vi "Jog Move.vi"(4 "Stop Move":bool, 5 "Error In":errorcluster, 6 "Velocity [rev/s]":dbl(knob)=1000.0 scale=0.0..10.0, 7 "Position Limit [deg]":dbl=1000.0, 8 "Resource in":refnum<k21>="Axis 1") -> (0 "Move Position":dbl(graph), 1 "Jogging":bool, 2 "error out":errorcluster, 3 "Resource out":refnum<k21>="Axis 1")   [LabVIEW 2018]
uses:
  <vilib>/Motion/Express/_s/nimc.ex.clearFaults.clearFaults.axis.vi
  <vilib>/Motion/Express/_s/nimc.ex.read.readExecutionData.axis.vi
  <vilib>/Motion/Express/_s/nimc.ex.stopMove.stop.axis.modeDecelerate.vi
  <vilib>/Motion/Express/_s/nimc.ex.straightLineMove.startStraightLineMove.axis.modeAbsolute.0.vi
  <vilib>/Motion/BlockNode/FB.NIMotion.xnode
panel:
  out "Jog done":bool
  # "INPUTS"
  # "Stop Move"
  # "OUTPUTS"
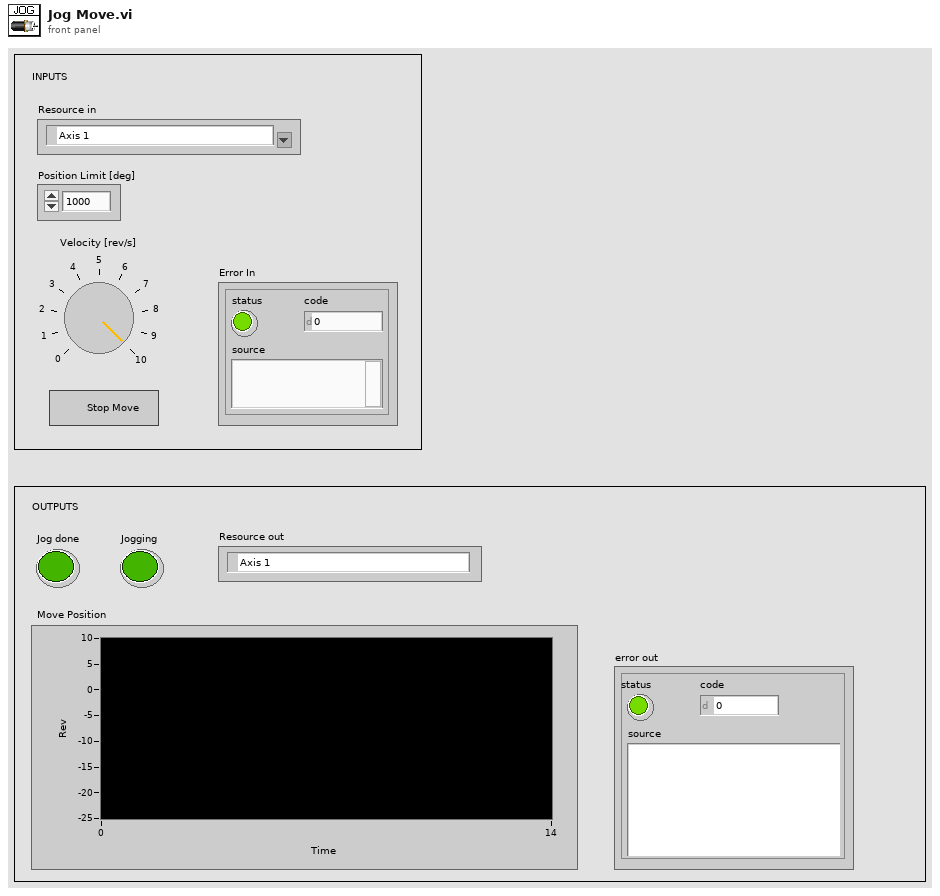
[diagram p1: front panel]
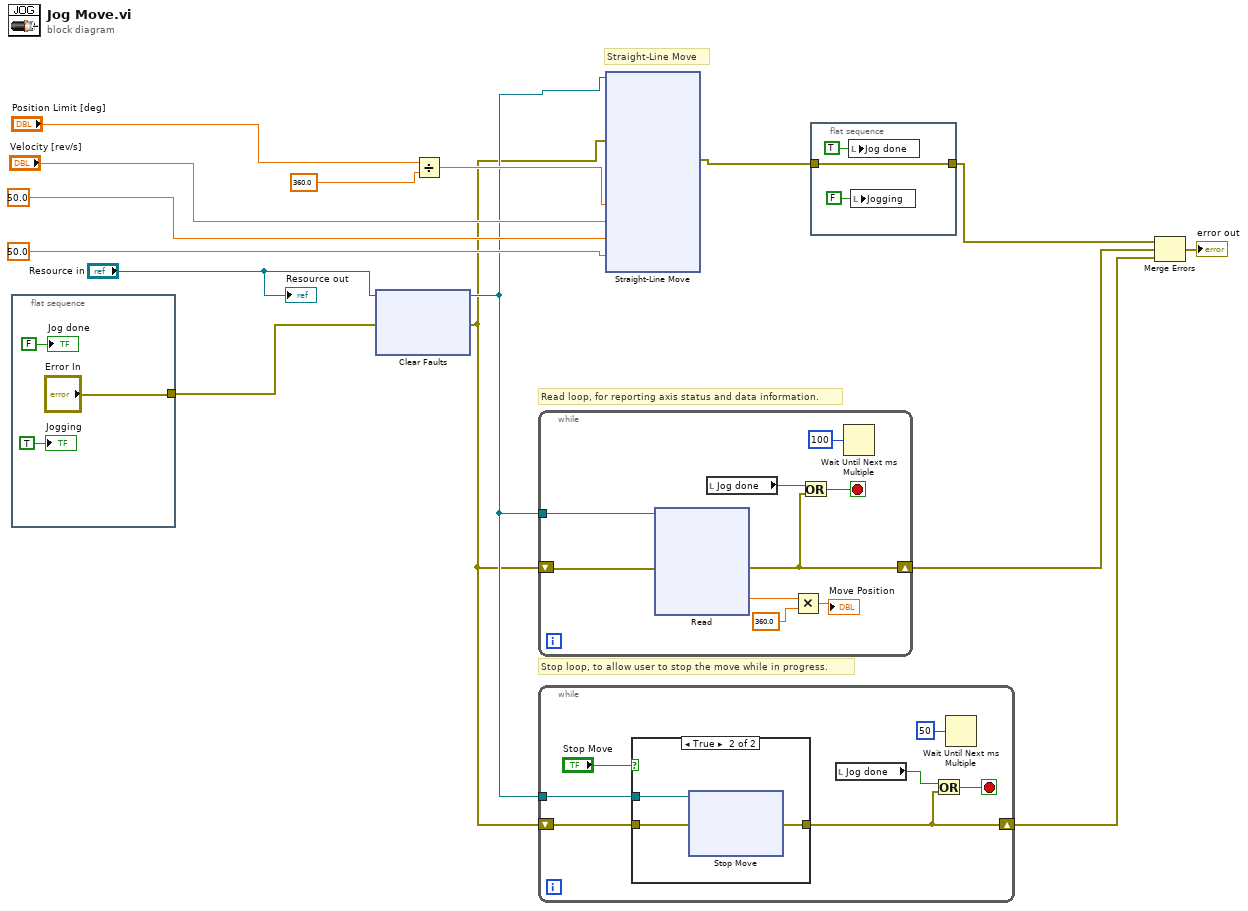
[diagram p0: block diagram]
diagram:
  # "Read loop, for reporting axis status and data information."
  # "Stop loop, to allow user to stop the move while in progress."
  # "Straight-Line Move"
  n1 = flat-sequence {
    tunnel: ["Error In"] -> w12
    frame #0 {
      "Jog done" <- FALSE ("Example Done")
      "Jogging" <- TRUE ("Example Done")
    }
  }
  n2 = xnode ("Clear Faults")("resource"="Resource in", "error in"=w12) -> ("resource out"=w4:refnum<k21>, "error out"=w1:errorcluster)
  n3 = Divide(x="Position Limit [deg]", y=360.0) -> (x/y=w5:dbl)
  n4 = while {
    tunnel: w4 -> [w25]
    shift-right: [w24] -> w14
    shift-left: w1 -> [w22]
    stop <- w27 stop-if-true
    n5 = xnode ("Read")("resource"=w25, "error in"=w22) -> ("position"=w21:dbl, "error out"=w24:errorcluster)  [unwired: 5 out]
    n6 = local read "Jog done"() -> (w26:bool)
    n7 = Multiply(x=w21, y=360.0) -> (x*y=→"Move Position":dbl)
    n8 = Or(x=w26, y=w24) -> (x .or. y?=w27:bool)
    n9 = Wait Until Next ms Multiple(millisecond multiple=u32 100) -> ()  [unwired: 1 out]
  }
  n10 = while {
    tunnel: w4 -> [w41]
    shift-right: [w39] -> w13
    shift-left: w1 -> [w40]
    stop <- w37 stop-if-true
    n11 = case shown="True" "Stop Move" {
      tunnel: [w44 w47] -> w39
      tunnel: w41 -> [_ w46]
      tunnel: w40 -> [w44 w45]
      frame False {
      }
      frame True {
        n12 = xnode ("Stop Move")("resource"=w46, "error in"=w45) -> ("error out"=w47:errorcluster)  [unwired: 1 in, 2 out]
      }
    }
    n13 = local read "Jog done"() -> (w38:bool)
    n14 = Or(x=w38, y=w39) -> (x .or. y?=w37:bool)
    n15 = Wait Until Next ms Multiple(millisecond multiple=u32 50) -> ()  [unwired: 1 out]
  }
  n16 = xnode ("Straight-Line Move")("position"=w5, "velocity"="Velocity [rev/s]", "deceleration"=50.0, "decel. jerk"=50.0, "resource"=w4, "error in"=w1) -> ("error out"=w3:errorcluster)  [unwired: 4 in, 2 out]
  n17 = flat-sequence {
    tunnel: w3 -> [w58]
    tunnel: [w58] -> w2
    frame #0 {
      n18 = local write "Jog done"(TRUE ("Jog done")) -> ()
      n19 = local write "Jogging"(FALSE ("Jogging")) -> ()
    }
  }
  n20 = Merge Errors(w2, w14, w13) -> (→"error out":errorcluster)
  "Resource out" <- "Resource in"
